vi "SetSourceFormat.vi"(8 "Error In":errorcluster, 10 "Source Format":T1, 11 "Keithley 6482 In":refnum<visa-resource-name>) -> (0 "Error Out":errorcluster, 3 "Keithley 6482 Out":refnum<visa-resource-name>)   [LabVIEW 2012, in "Keithley-6482.lvlib"]
uses:
  Keithley-6482.lvlib
  Controls/SourceFormat.ctl
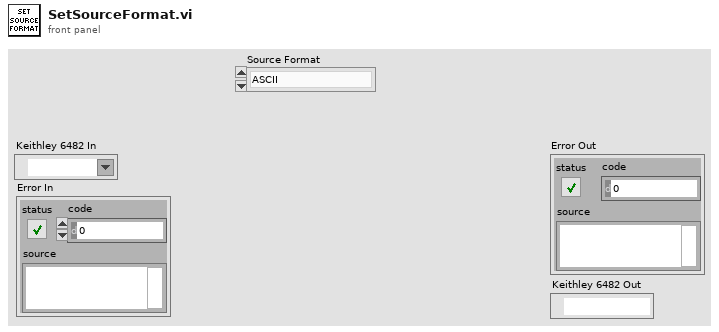
[diagram p1: front panel]
types:
  T1 = typedef "Keithley-6482.lvlib/SourceFormat.ctl" = enum16{"ASCII", "Hexadecimal", "Octal", "Binary"}
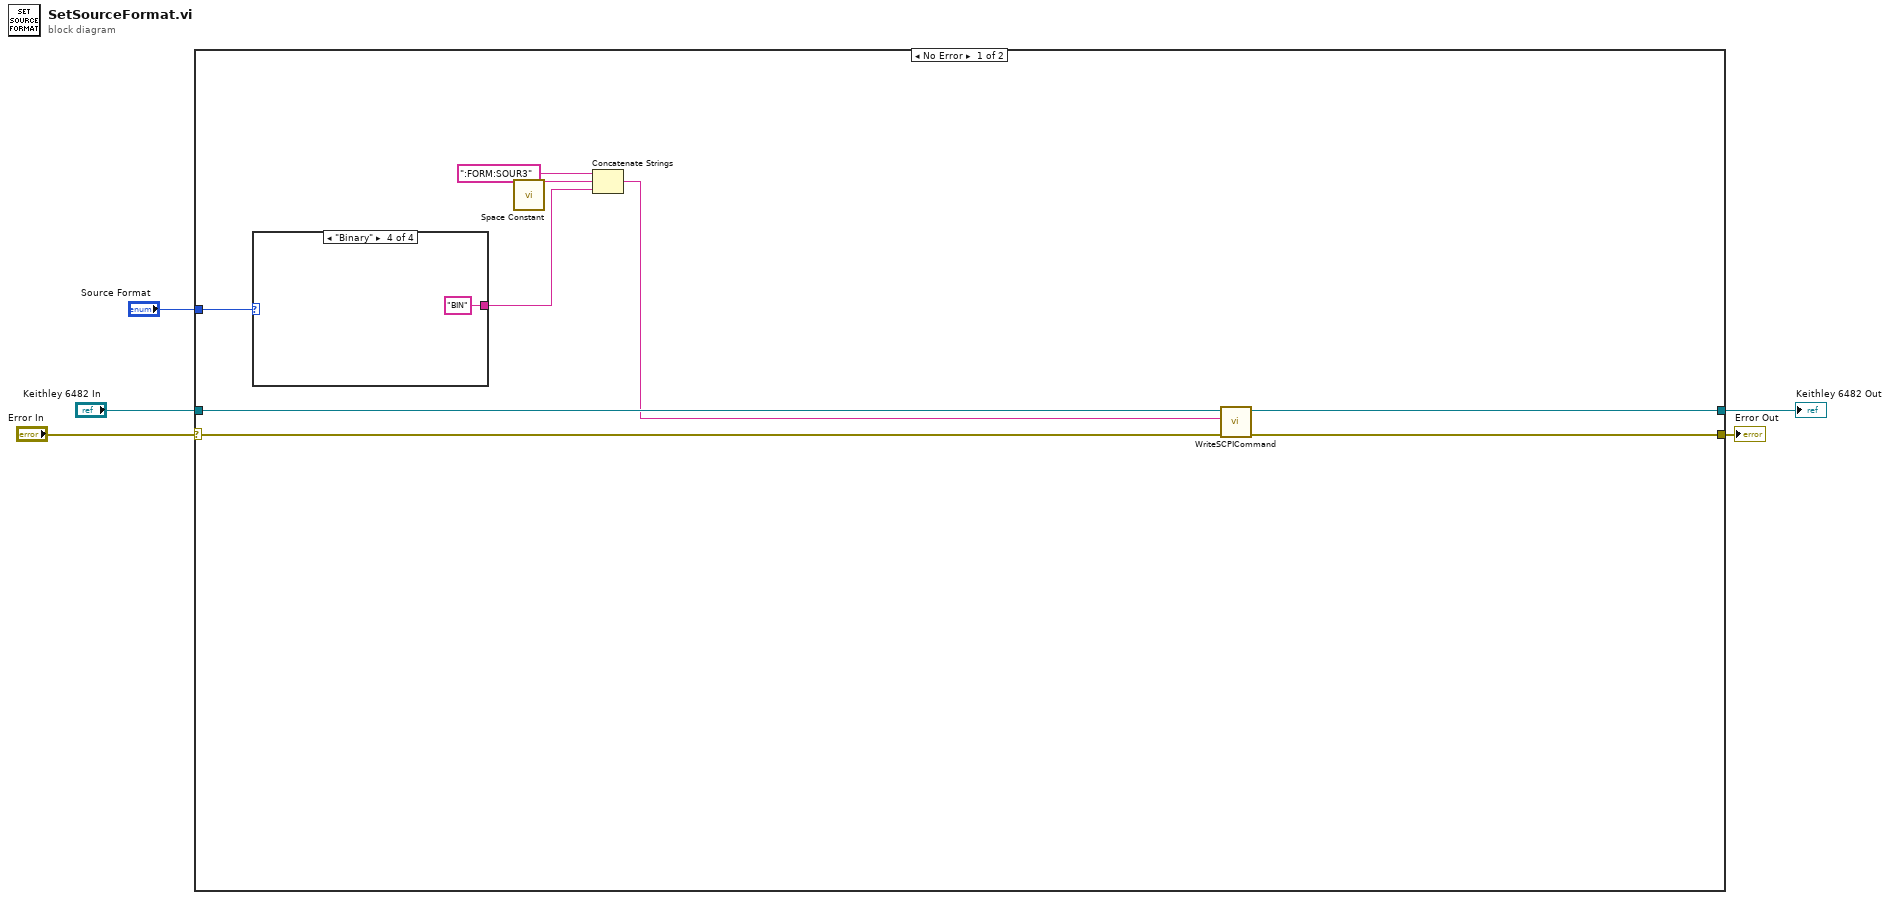
[diagram p0: block diagram]
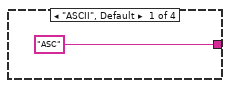
[diagram p2: hidden frame]
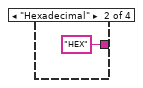
[diagram p3: hidden frame]
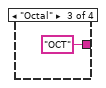
[diagram p4: hidden frame]
diagram:
  n1 = case shown="No Error" "Error In" {
    selector: "Error In" -> [w10 w19]
    tunnel: "Keithley 6482 In" -> [w9 w20]
    tunnel: [w11 w19] -> w3
    tunnel: [w12 w20] -> w2
    tunnel: "Source Format" -> [w7 _]
    frame No Error {
      n2 = case shown="\"Binary\"" w7 {
        tunnel: ["ASC" "HEX" "OCT" "BIN"] -> w6
        frame "ASCII", Default {
        }
        frame "Hexadecimal" {
        }
        frame "Octal" {
        }
        frame "Binary" {
        }
      }
      n3 = call <vilib>:"Space Constant.vi"() -> ("String"=w13:string)
      n4 = Concatenate Strings(":FORM:SOUR3", w13, w6) -> (w8:string)
      n5 = call "WriteSCPICommand.vi"("Error In"=w10, "SCPI Command"=w8, "Keithley 6482 In"=w9) -> ("Error Out"=w11:errorcluster, "Keithley 6482 Out"=w12:refnum<visa-resource-name>)  [unwired: 7 in]
    }
    frame Error {
    }
  }
  "Error Out" <- w3
  "Keithley 6482 Out" <- w2
